vi "Create Helium Test Page.vi"(7 "Data":string[][](array[string]), 8 "error in (no error)":errorcluster, 11 "Report In":refnum<class "NI_report.lvclass">) -> (0 "error out":errorcluster, 3 "Report Out":refnum<class "NI_report.lvclass">)   [LabVIEW 2014]
uses:
  <vilib>/Utility/NIReport.llb/NI_report.lvclass
  <vilib>/addons/_office/_exclsub.llb/font.ctl
  <vilib>/addons/_office/excel.llb/Excel Easy Table (str).vi
  <vilib>/addons/_office/NI_ReportGenerationToolkit.lvlib
  <vilib>/Utility/NIReport.llb/Excel/NI_Excel.lvclass
panel:
  in  "Start Cell":cluster{"row":i32, "column":i32}={"row"=3, "column"=0}
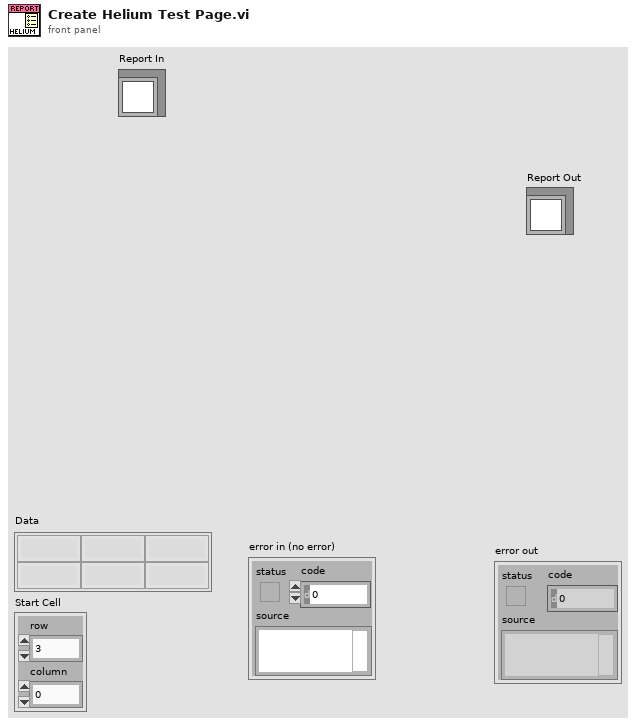
[diagram p1: front panel]
types:
  T1 = typedef "NI_ReportGenerationToolkit.lvlib/font.ctl" = cluster{"font name":string, "font size":dbl, "bold":u16, "italic":u16, "underline":u16, "strike through":u16, "font color":u32}
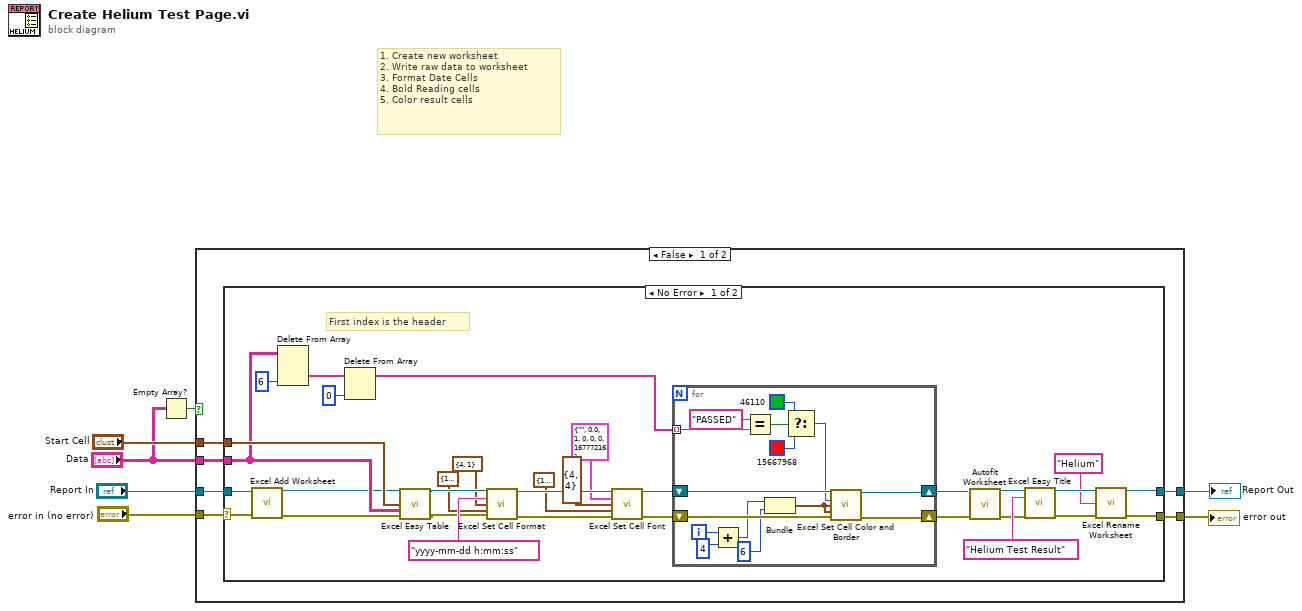
[diagram p0: block diagram]
diagram:
  # "1. Create new worksheet\n2. Write raw data to worksheet\n3. Format Date Cells\n4. Bold Reading cells\n5. Color result cells"
  n1 = Empty Array?(array="Data") -> (empty?=w1:bool)
  n2 = case shown="False" w1 {
    tunnel: [w13 w64] -> w7
    tunnel: "error in (no error)" -> [w12 w64]
    tunnel: "Report In" -> [w11 w63]
    tunnel: [w10 w63] -> w4
    tunnel: "Start Cell" -> [w9 _]
    tunnel: "Data" -> [w8 _]
    frame False {
      n3 = case shown="No Error" w12 {
        selector: w12 -> [w40 w62]
        tunnel: [w18 w62] -> w13
        tunnel: w11 -> [w41 w61]
        tunnel: [w17 w61] -> w10
        tunnel: w9 -> [w42 _]
        tunnel: w8 -> [w29 _]
        frame No Error {
          # "First index is the header"
          n4 = call <vilib>:"Excel Add Worksheet.vi"("report in"=w41, "error in (no error)"=w40) -> ("report out"=w15:refnum<class "NI_report.lvclass">, "error out"=w14:errorcluster)  [unwired: 12 in]
          n5 = Delete From Array(array=w29, index (col)=6 ("disabled index (col)")) -> (deleted portion=w27:string[])  [unwired: 2 in, 1 out]
          n6 = Delete From Array(array=w27, index=0) -> (array with subset deleted=w26:string[])  [unwired: 1 in, 1 out]
          n7 = call-poly <vilib>:"Excel Easy Table.vi"("report in"=w15, "start (0, 0)"=w42, "text data"=w29, "error in (no error)"=w14) -> ("report out"=w38:refnum<class "NI_report.lvclass">, "error out"=w37:errorcluster)  [unwired: 7 in, 3 out]
          n8 = call <vilib>:"Excel Set Cell Format.vi"("report in"=w38, "number format"="yyyy-mm-dd h:mm:ss", "start (-1, -1)"=cluster{"row":i32, "column":i32} {"row"=4, "column"=1}, "end (-1, -1)"=cluster{"row":i32, "column":i32} {"row"=100, "column"=2} ("start (-1, -1)"), "error in (no error)"=w37) -> ("report out"=w34:refnum<class "NI_report.lvclass">, "error out"=w33:errorcluster)  [unwired: 9 in]
          n9 = call <vilib>:"Excel Set Cell Font.vi"("report in"=w34, "font"=T1 {"font name"="", "font size"=0.0, "bold"=1, "italic"=0, "underline"=0, "strike through"=0, "font color"=16777216}, "start (-1, -1)"=cluster{"row":i32, "column":i32} {"row"=4, "column"=4}, "end (-1, -1)"=cluster{"row":i32, "column":i32} {"row"=100, "column"=4} ("start (-1, -1)"), "error in (no error)"=w33) -> ("report out"=w22:refnum<class "NI_report.lvclass">, "error out"=w21:errorcluster)  [unwired: 9 in]
          n10 = for {
            tunnel: w26 -> [w60] mode=indexing
            shift-right: [w46] -> w24
            shift-left: w22 -> [w55]
            shift-right: [w52] -> w23
            shift-left: w21 -> [w53]
            i -> [w51]
            n11 = Add(x=w51, y=4) -> (x+y=w49:i32)
            n12 = Equal?(x="PASSED", y=w60) -> (x = y?=w58:bool)
            n13 = Bundle(w49, "y"=6) -> (w47:cluster{i32, "y":i32})  [unwired: 1 in]
            n14 = Select(t=u32 46110, s=w58, f=u32 15667968) -> (s? t:f=w54:u32)
            n15 = call <vilib>:"Excel Set Cell Color and Border.vi"("report in"=w55, "background color (w)"=w54, "start (-1, -1)"=w47, "end (-1, -1)"=w47, "error in (no error)"=w53) -> ("report out"=w46:refnum<class "NI_report.lvclass">, "error out"=w52:errorcluster)  [unwired: 9 in]
          }
          n16 = call "Autofit Worksheet.vi"("error in (no error)"=w23, "Report In"=w24) -> ("error out"=w43:errorcluster, "Report Out"=w44:refnum<class "NI_report.lvclass">)  [unwired: 8 in]
          n17 = call <vilib>:"Excel Easy Title.vi"("report in"=w44, "title"="Helium Test Result", "error in (no error)"=w43) -> ("report out"=w20:refnum<class "NI_report.lvclass">, "error out"=w19:errorcluster)  [unwired: 10 in, 1 out]
          n18 = call <vilib>:"Excel Rename Worksheet.vi"("report in"=w20, "worksheet name (\"\")"="Helium" ("worksheet name (\"\")"), "error in (no error)"=w19) -> ("report out"=w17:refnum<class "NI_report.lvclass">, "error out"=w18:errorcluster)  [unwired: 11 in]
        }
        frame Error {
        }
      }
    }
    frame True {
    }
  }
  "error out" <- w7
  "Report Out" <- w4
